vi "Configure Remote Trace Autoscroll Enabled.vi"(8 "error in (no error)":errorcluster, 10 "Autoscroll (On)":bool=TRUE, 11 "VISA resource name":refnum<visa-resource-name>) -> (0 "error out":errorcluster, 3 "VISA resource name out":refnum<visa-resource-name>)   [LabVIEW 2020, in "Rohde&Schwarz CMXP Base.lvlib"]
doc: "Enables automatic scrolling for the trace log on the screen.\n\nAttribute:\nRSCMXPBASE_ATTR_REMOTE_TRACE_AUTOSCROLL_ENABLED\n\nRemote-control command:\n[CONFigure:]BASE:RTRace:ASCRoll"
uses:
  <instrlib>/Rohde&Schwarz CMXP Base/Rohde&Schwarz CMXP Base.lvlib
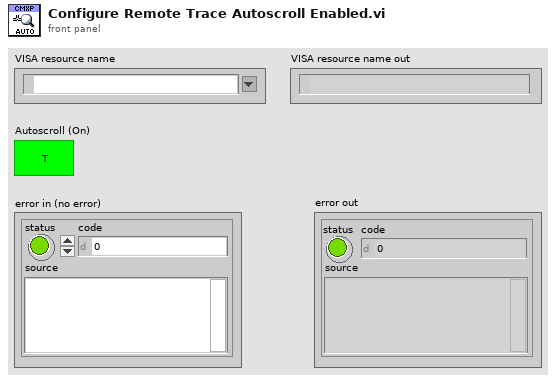
[diagram p1: front panel]
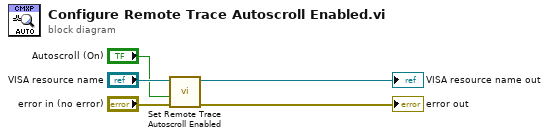
[diagram p0: block diagram]
diagram:
  n1 = call "Set Remote Trace Autoscroll Enabled"("error in (no error)"="error in (no error)", "Remote Trace Autoscroll Enabled (OFF)"="Autoscroll (On)", "instrument handle"="VISA resource name") -> ("error out"=→"error out":errorcluster, "instrument handle out"=→"VISA resource name out":refnum<visa-resource-name>)  [unwired: 7 in]
